vi "Process 2.vi"(11 "PROC1-USER EVENTS":T1) -> ()   [LabVIEW 2014]
panel:
  out "error out":errorcluster
  in  "error in (no error)":errorcluster
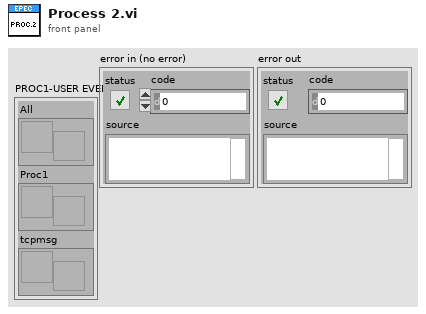
[diagram p1: front panel]
types:
  T1 = cluster{"All":refnum<user-event>, "Proc1":refnum<user-event>, "tcpmsg":refnum<user-event>}
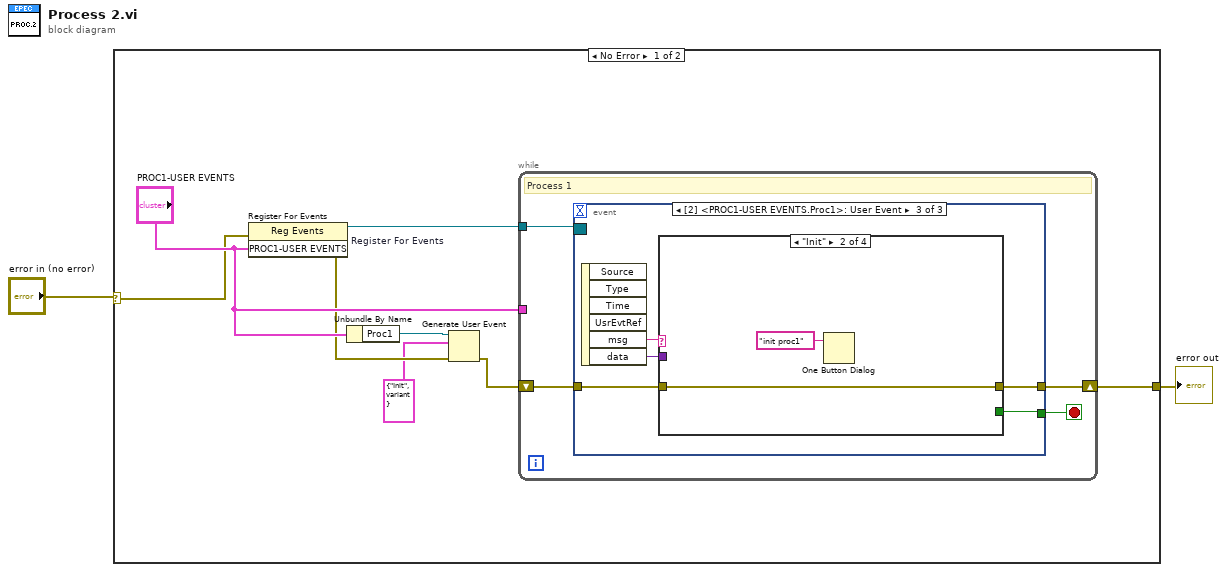
[diagram p0: block diagram]
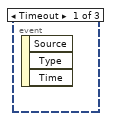
[diagram p2: hidden frame]
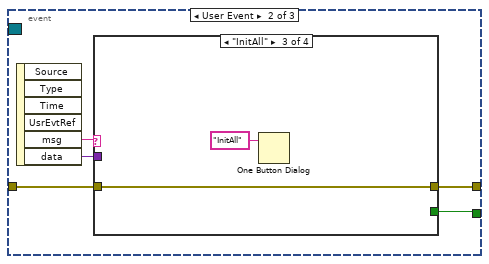
[diagram p3: hidden frame]
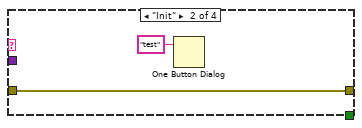
[diagram p5: hidden frame]
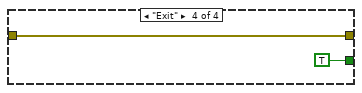
[diagram p6: hidden frame]
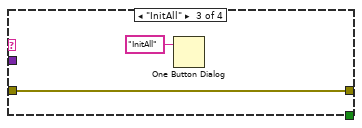
[diagram p8: hidden frame]
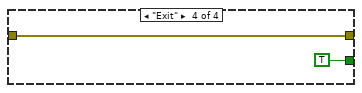
[diagram p9: hidden frame]
diagram:
  n1 = case shown="No Error" "error in (no error)" {
    selector: "error in (no error)" -> [w4 w39]
    tunnel: [w3 w39] -> w1
    frame No Error {
      n2 = register-events "Register For Events"(error in=w4, "PROC1-USER EVENTS") -> (reference out=w5:refnum<event-registration>, error out=w7:errorcluster)  [unwired: 1 in]
      n3 = Unbundle By Name("PROC1-USER EVENTS") -> ("Proc1"=w10:refnum<user-event>)
      n4 = Generate User Event(user event=w10, event data cluster=cluster{"msg":string, "data":variant} {"msg"="Init", "data"=variant} ("event data"), error in=w7) -> (error out=w8:errorcluster)  [unwired: 1 in, 1 out]
      n5 = while {
        tunnel: w5 -> [w13]
        shift-right: [w11] -> w3
        shift-left: w8 -> [w12]
        tunnel: "PROC1-USER EVENTS" -> [_]
        stop <- w14 stop-if-true
        # "Process 1"
        n6 = event shown="[2] <PROC1-USER EVENTS.Proc1>: User Event" {
          selector: w13 -> [_ _ _]
          dyn-events: _ -> [_ _ _]
          timeout: _ -> [_ _ _]
          tunnel: [_ w17 w29] -> w14
          tunnel: w12 -> [_ w16 w28]
          tunnel: [_ w15 w27] -> w11
          event Timeout {
            n7 = event-data() -> ()  [unwired: 1 in, 3 out]
          }
          event User Event {
            n8 = event-data() -> ("msg"=w19:string, "data"=w18:variant)  [unwired: 1 in, 4 out]
            n9 = case shown="\"InitAll\"" w19 {
              tunnel: w18 -> [_ _ _ _]
              tunnel: [_ _ _ TRUE ("stop 2")] -> w17
              tunnel: w16 -> [w20 w22 w24 w25]
              tunnel: [w20 w22 w24 w25] -> w15
              frame Default {
              }
              frame "Init" {
                n10 = One Button Dialog(message="test") -> ()  [unwired: 1 in, 1 out]
              }
              frame "InitAll" {
                n11 = One Button Dialog(message="InitAll") -> ()  [unwired: 1 in, 1 out]
              }
              frame "Exit" {
              }
            }
          }
          event User Event {
            n12 = event-data() -> ("msg"=w31:string, "data"=w30:variant)  [unwired: 1 in, 4 out]
            n13 = case shown="\"Init\"" w31 {
              tunnel: w30 -> [_ _ _ _]
              tunnel: [_ _ _ TRUE ("stop 2")] -> w29
              tunnel: w28 -> [w32 w34 w36 w37]
              tunnel: [w32 w34 w36 w37] -> w27
              frame Default {
              }
              frame "Init" {
                n14 = One Button Dialog(message="init proc1") -> ()  [unwired: 1 in, 1 out]
              }
              frame "InitAll" {
                n15 = One Button Dialog(message="InitAll") -> ()  [unwired: 1 in, 1 out]
              }
              frame "Exit" {
              }
            }
          }
        }
      }
    }
    frame Error {
    }
  }
  "error out" <- w1
